vi "Master_DAQ_fixPT.vi"(1 "new value":dbl) -> (0 "mean":dbl format="%0.2f")   [LabVIEW 2017]
uses:
  <vilib>/Analysis/baseanly.llb/Mean (DBL).vi
  <vilib>/addons/Time Series Analysis/Series Preprocess.llb/TSA Moving Average (Array).vi
  <vilib>/Analysis/NI_AALBase.lvlib
  <vilib>/addons/_Advanced Signal Processing/NI_AdvSigProcTSA.lvlib
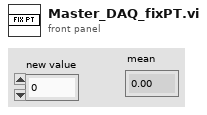
[diagram p1: front panel]
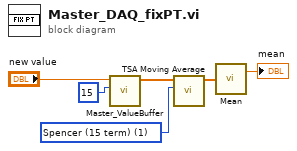
[diagram p0: block diagram]
diagram:
  w1 = 1 items=["Spencer (15 term)"=1, "Henderson (7 term)"=2, "Henderson (9 term)"=3, "Henderson (13 term)"=4, "Henderson (23 term)"=5] ("method")
  n1 = call "Master_ValueBuffer.vi"("n"=15, "new value"="new value") -> ("Last n values"=w2:dbl[])  [unwired: 9 in]
  n2 = call-poly <vilib>:"TSA Moving Average.vi"("method"=w1, "Xt"=w2) -> ("Xt out"=w4:dbl[])  [unwired: 8 in, 1 out]
  n3 = call-poly <vilib>:"Mean.vi"("X"=w4) -> ("mean"=→"mean":dbl)  [unwired: 1 out]
